vi "Subvi AO Pockels.vi"(2 "AO":refnum<k21>="Connector1/AO0", 8 "Scaling Factor":refnum<k21>="SCALING1", 9 "FIFO":refnum<k21>="POCKELS1") -> ()   [LabVIEW 2017]
uses:
  <vilib>/Platform/TimedLoop/XDataNode/timing_clust.ctl
  <vilib>/Platform/TimedLoop/XDataNode/nitl_modes.ctl
  <vilib>/Platform/TimedLoop/XDataNode/wakeup.ctl
  <vilib>/rvi/Emulation/niFpgaSctlEmulationGetInTimedLoop.vi
  <vilib>/rvi/Emulation/niFpgaEmulationReportErrorSimple.vi
  <vilib>/rvi/Emulation/niFpgaGetClockAttributes.vi
  <vilib>/rvi/Emulation/niFpgaCriticalErrorInLSC.vi
  GV preframeclock.vi
  GV frame counter.vi
  <vilib>/rvi/DataTransferAndStorage/Container/Common/niFpgaContainerExecOnDevCompGetState.vi
  <vilib>/rvi/Emulation/niFpgaEmulationIsFPGAContextNoSignature.vi
  <vilib>/rvi/DataTransferAndStorage/Container/Common/niFpgaContainerGetUniqueNameForEmu.vi
  <vilib>/rvi/Emulation/niFpgaProcessEmulError.vi
  <vilib>/rvi/errors/nirviReportUnexpectedCaseInternalError (U32).vi
  <vilib>/rvi/Memory/Memory_Emulation/niFpgaMemoryEmulationCacheClearOnFirstRun.vi
  <vilib>/rvi/Memory/Memory_Emulation/nirvimemoryEmulationManagerCache_MakeExclusive.vi
  <vilib>/rvi/Memory/Memory_Emulation/niFpgaMemoryEmulationValidateCache.vi
  <vilib>/rvi/Memory/Memory_Emulation/nirvimemoryEmulationManagerCache_InsertValue.vi
  <vilib>/Utility/error.llb/Clear Errors.vi
  <vilib>/rvi/Memory/Memory_Emulation/nirvimemoryEmulationManagerCache_ReleaseExclusive.vi
  <vilib>/rvi/Memory/Memory_Emulation/nirvimemoryEmulationManagerCache_GetValue.vi
  <vilib>/rvi/Memory/Memory_Emulation/nirvimemoryEmulationManagerCache_SetValue.vi
  <vilib>/rvi/Emulation/niFpgaSctlEmulationResourceMgr.vi
  <vilib>/rvi/eio/common/nirviEmuTemplateMethod_errors.vi
  <vilib>/Platform/TimedLoop/XDataNode/XDataNode.xnode
  <vilib>/rvi/DataTransferAndStorage/Container/XNode/niFpgaContainer.xnode
  <vilib>/rvi/Memory/Memory_Emulation/niFpgaMemoryEmulationRefIn.vi
  <vilib>/eio/EIONode/EIONode.xnode
  <vilib>/Platform/TimedLoop/XDataNode/XDNodeRunTimeDep.lvlib
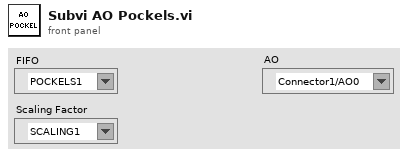
[diagram p1: front panel]
types:
  T1 = typedef "XDNodeRunTimeDep.lvlib/timing_clust.ctl" = cluster{"Expected End [f-1]":u64, "Actual End [f-1]":u64, "Finished Late? [f-1]":bool, "Expected End [i-1]":u64, "Actual End [i-1]":u64, "Finished Late? [i-1]":bool, "Expected Start [i]":u64, "Actual Start [i]":u64, "Expected Start [f]":u64, "Actual Start [f]":u64, "Source Name":string, "Structure Name":string, "Period":i64, "Deadline":i64, "Offset":i64, "Start":i64, "Priority":i32, "Timeout":i32, "Mode":T2, "Wakeup Reason":T3, "Error":errorcluster, "Source Type":string, "Secondary Source Type":string, "Global End Time":u64, "Global Start Time":u64, "Frame Duration":u64, "Iteration Duration":u64, "Assigned CPU":i32, "I/O Scan Engine Mode":u32}
  T2 = typedef "XDNodeRunTimeDep.lvlib/nitl_modes.ctl" = enum32{"No Change", "Process missed periods, maintain original phase", "Discard missed periods, maintain original phase", "Process missed periods, ignore original phase", "Discard missed periods, ignore original phase"}
  T3 = typedef "XDNodeRunTimeDep.lvlib/wakeup.ctl" = enum32{"Normal", "Aborted", "Asynchronous wakeup", "Timing source error", "Timed loop error", "Timeout"}
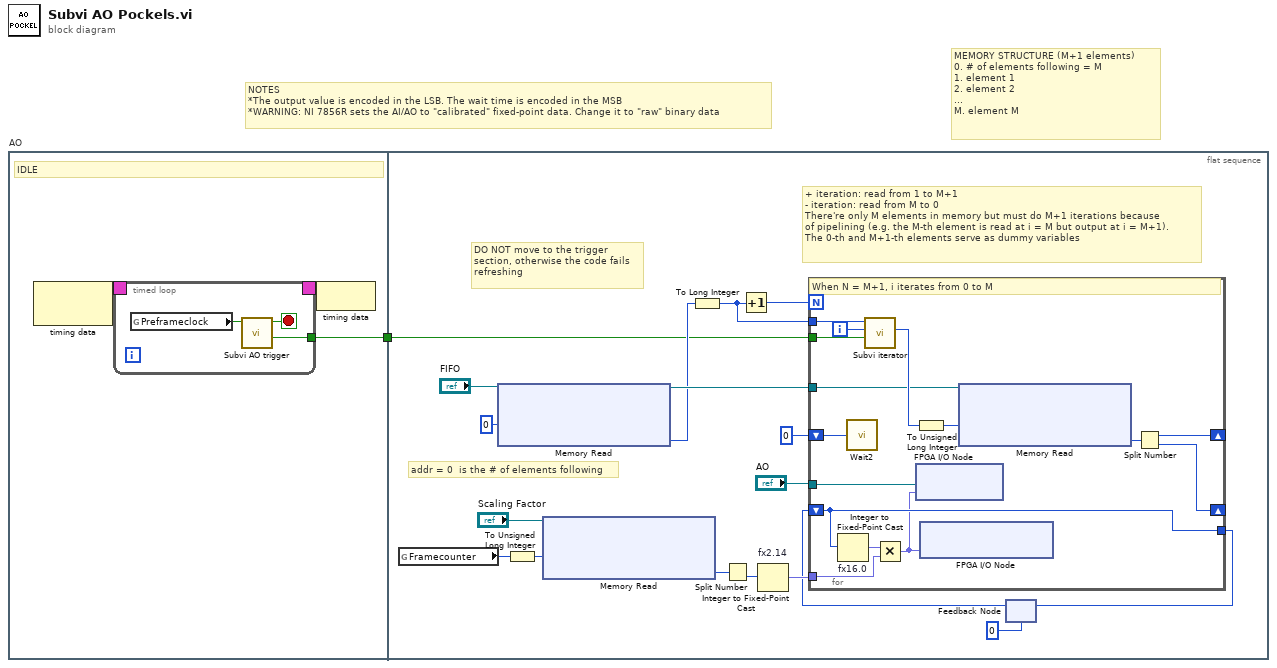
[diagram p0: block diagram]
diagram:
  # "MEMORY STRUCTURE (M+1 elements)\n0. # of elements following = M\n1. element 1\n2. element 2\n...\nM. element M"
  # "NOTES\n*The output value is encoded in the LSB. The wait time is encoded in the MSB\n*WARNING: NI 7856R sets the AI/AO to \"calibrated\" fixed-point data. Change it to \"raw\" binary data"
  n1 = flat-sequence "AO" {
    tunnel: [w4] -> w1
    tunnel: w1 -> [w12]
    frame #0 {
      # "IDLE"
      n2 = node-c288() -> (w3:T1)  [unwired: 1 in]
      n3 = timed-loop {
        timing: w3 -> [_]
        timing-out: [_] -> w2
        tunnel: [w5] -> w4
        stop <- w6 stop-if-true
        n4 = global read "GV preframeclock.vi" "Preframeclock"() -> (w7:bool)
        n5 = call "Subvi AO trigger.vi"("Frameclock"=w7) -> ("IteratorDirection"=w5:bool, "Stop"=w6:bool)  [unwired: 9 in]
      }
      n6 = node-c288(w2) -> ()
    }
    frame #1 {
      # "+ iteration: read from 1 to M+1\n- iteration: read from M to 0\nThere're only M elements in memory but must do M+1 iterations because \nof pipelining (e.g. the M-th element is read at i = M but output at i = M+1).\nThe 0-th and M+1-th elements serve as dummy variables"
      # "addr = 0  is the # of elements following"
      # "DO NOT move to the trigger\nsection, otherwise the code fails\nrefreshing"
      n7 = global read "GV frame counter.vi" "Framecounter"() -> (w16:u8)
      n8 = xnode ("Memory Read")("Address"=u32 0, "Memory In"="FIFO") -> ("Data"=w18:u32, "Memory Out"=w28:refnum<k21>)
      n9 = To Unsigned Long Integer(number=w16) -> (unsigned 32bit integer=w20:u32)
      n10 = xnode ("Memory Read")("Address"=w20, "Memory In"="Scaling Factor") -> ("Data"=w22:u32)  [unwired: 1 out]
      n11 = To Long Integer(number=w18) -> (32bit integer=w17:i32)
      n12 = Split Number(x=w22) -> (lo(x)=w25:u16)  [unwired: 1 out]
      n13 = Increment(x=w17) -> (x+1=w19:i32)
      n14 = Integer to Fixed-Point Cast "fx2.14"(integer=w25) -> (fixed-point=w24:fxp<+,16,2>)  [unwired: 1 in]
      n15 = feedback #1(u16 0) -> (w14:u16)
      n16 = for {
        N: w19 -> [_]
        shift-right: [w42] -> _
        shift-left: u16 0 -> [w41]
        shift-right: [w31] -> _
        shift-left: w14 -> [w34]
        tunnel: [w34] -> w15
        tunnel: w17 -> [w38]
        tunnel: w28 -> [w37]
        tunnel: w12 -> [w36]
        tunnel: w24 -> [w35]
        tunnel: "AO" -> [w30]
        i -> [w39]
        # "When N = M+1, i iterates from 0 to M"
        n17 = Integer to Fixed-Point Cast "fx16.0"(integer=w34) -> (fixed-point=w33:fxp<+/-,16,16>)  [unwired: 1 in]
        n18 = call "Wait2"("Count(Ticks)"=w41) -> ()  [unwired: 1 out]
        n19 = call "Subvi iterator.vi"("Set increase"=w36, "Iterator in"=w39, "Nmax"=w38) -> ("Iterator out"=w40:i32)  [unwired: 8 in]
        n20 = Multiply(x=w33, y=w35) -> (x*y=w32:fxp<+/-,32,18>)
        n21 = To Unsigned Long Integer(number=w40) -> (unsigned 32bit integer=w44:u32)
        n22 = xnode ("FPGA I/O Node")("I/O Item"=w32, "FPGA I/O In"=w30) -> ()  [unwired: 1 out]
        n23 = xnode "FPGA I/O Node"("Connector1/AO7"=w32) -> ()  [unwired: 1 in, 1 out]
        n24 = xnode ("Memory Read")("Address"=w44, "Memory In"=w37) -> ("Data"=w43:u32)  [unwired: 1 out]
        n25 = Split Number(x=w43) -> (hi(x)=w42:u16, lo(x)=w31:u16)
      }
      n26 = feedback-in #1(w15) -> ()
    }
  }
